vi "resize window.vi"(10 "parameters":variant[](array[variant]), 11 "vis":refnum<vi>[](array[refnum])) -> (0 "error report":errorcluster[](array[cluster]))   [LabVIEW 2013]
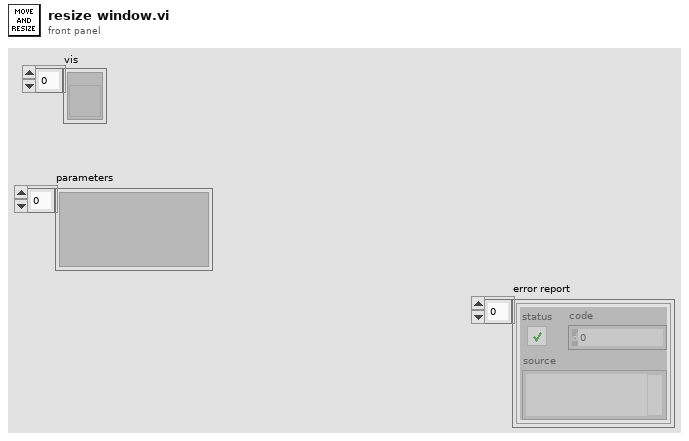
[diagram p1: front panel]
types:
  T1 = typedef "LVRectTypeDef.ctl" = cluster{"Left":i16, "Top":i16, "Right":i16, "Bottom":i16}
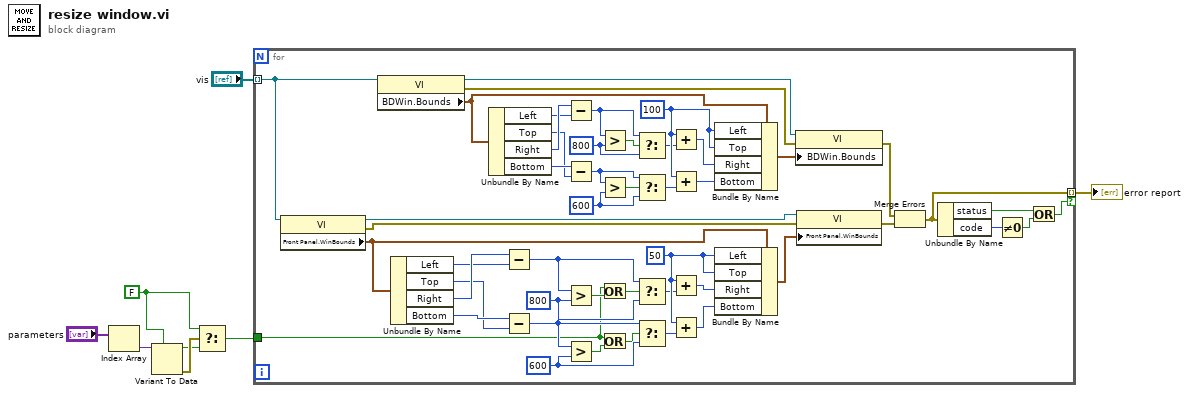
[diagram p0: block diagram]
diagram:
  w3 = FALSE
  n1 = Index Array(array="parameters") -> (element=w5:variant)  [unwired: 1 in]
  n2 = Variant To Data(type=w3, Variant=w5) -> (data=w2:bool, error out=w4:errorcluster)  [unwired: 1 in]
  n3 = Select(t=w3, s=w4, f=w2) -> (s? t:f=w1:bool)
  n4 = for {
    tunnel: "vis" -> [w13] mode=indexing
    tunnel: [w9] -> w7 mode=indexing if=w54
    tunnel: w1 -> [w12]
    w41 = i16 600 ("y")
    w40 = i16 800 ("y")
    w46 = i16 600 ("y")
    w47 = i16 800 ("y")
    w30 = i16 50 ("Left")
    w31 = i16 100 ("Left")
    n5 = property class="VI"(reference=w13) -> (reference out=w21:refnum<vi>, error out=w20:errorcluster, "Front Panel.WinBounds"=w16:T1)  [unwired: 1 in]
    n6 = property class="VI"(reference=w13) -> (reference out=w52:refnum<vi>, error out=w53:errorcluster, "BDWin.Bounds"=w19:T1)  [unwired: 1 in]
    n7 = Unbundle By Name(w16) -> ("Left"=w36:i16, "Top"=w32:i16, "Right"=w37:i16, "Bottom"=w33:i16)
    n8 = Unbundle By Name(w19) -> ("Left"=w50:i16, "Top"=w34:i16, "Right"=w51:i16, "Bottom"=w35:i16)
    n9 = Subtract(x=w37, y=w36) -> (x-y=w39:i16)
    n10 = Subtract(x=w33, y=w32) -> (x-y=w42:i16)
    n11 = Subtract(x=w51, y=w50) -> (x-y=w48:i16)
    n12 = Subtract(x=w35, y=w34) -> (x-y=w45:i16)
    n13 = Greater?(x=w39, y=w40) -> (0:w38:bool)
    n14 = Greater?(x=w42, y=w41) -> (0:w43:bool)
    n15 = Greater?(x=w48, y=w47) -> (0:w49:bool)
    n16 = Greater?(x=w45, y=w46) -> (0:w44:bool)
    n17 = Or(x=w12, y=w38) -> (x .or. y?=w15:bool)
    n18 = Or(x=w12, y=w43) -> (x .or. y?=w14:bool)
    n19 = Select(t=w48, s=w49, f=w47) -> (s? t:f=w26:i16)
    n20 = Select(t=w45, s=w44, f=w46) -> (s? t:f=w27:i16)
    n21 = Select(t=w39, s=w15, f=w40) -> (s? t:f=w29:i16)
    n22 = Select(t=w42, s=w14, f=w41) -> (s? t:f=w28:i16)
    n23 = Add(x=w31, y=w26) -> (x+y=w25:i16)
    n24 = Add(x=w31, y=w27) -> (x+y=w24:i16)
    n25 = Add(x=w30, y=w29) -> (x+y=w23:i16)
    n26 = Add(x=w30, y=w28) -> (x+y=w22:i16)
    n27 = Bundle By Name(cluster=w19, "Left"=w31, "Top"=w31, "Right"=w25, "Bottom"=w24) -> (w18:T1)
    n28 = Bundle By Name(cluster=w16, "Left"=w30, "Top"=w30, "Right"=w23, "Bottom"=w22) -> (w17:T1)
    n29 = property class="VI"(reference=w52, error in=w53, "BDWin.Bounds"=w18) -> (error out=w11:errorcluster)  [unwired: 1 out]
    n30 = property class="VI"(reference=w21, error in=w20, "Front Panel.WinBounds"=w17) -> (error out=w10:errorcluster)  [unwired: 1 out]
    n31 = Merge Errors(w11, w10) -> (w9:errorcluster)
    n32 = Unbundle By Name(w9) -> ("status"=w57:bool, "code"=w56:i32)
    n33 = Not Equal To 0?(x=w56) -> (x != 0?=w55:bool)
    n34 = Or(x=w57, y=w55) -> (x .or. y?=w54:bool)
  }
  "error report" <- w7
